vi "Write then read.vi"(7 "error in (no error)":errorcluster, 9 "TX Data":string, 10 "Motor_Serial in":refnum<class "Serial.lvclass">) -> (0 "error out":errorcluster, 2 "RX Data":i32, 3 "Motor_Serial out":refnum<class "Serial.lvclass">)   [LabVIEW 2019, in "Serial.lvclass"]
uses:
  Serial.lvclass
  Serial.lvclass/Serial.ctl
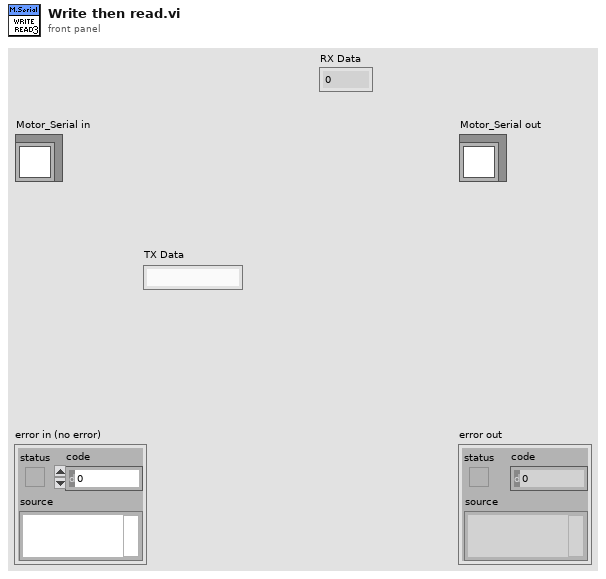
[diagram p1: front panel]
types:
  T1 = typedef "Semaphore RefNum" = refnum<k1>
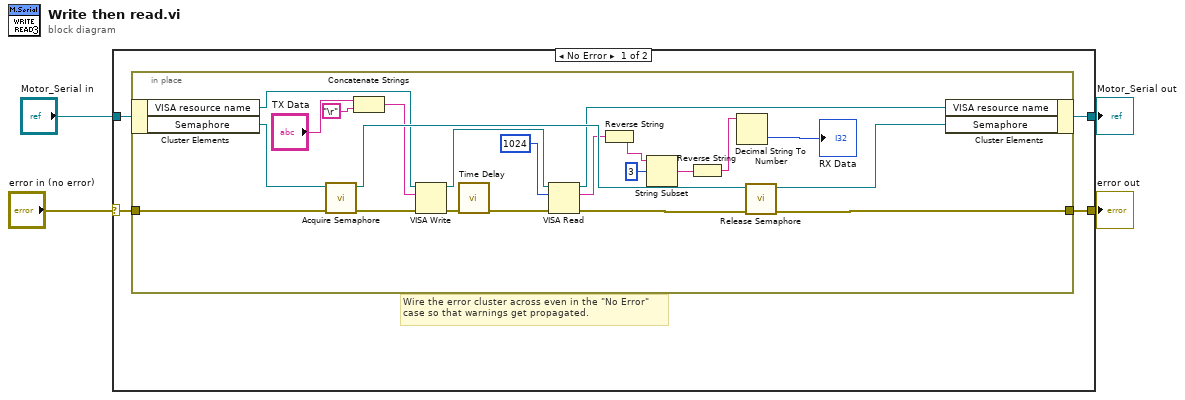
[diagram p0: block diagram]
diagram:
  n1 = case shown="No Error" "error in (no error)" {
    selector: "error in (no error)" -> [w8 w32]
    tunnel: [w7 w32] -> w3
    tunnel: [w5 w31] -> w1
    tunnel: "Motor_Serial in" -> [w6 w31]
    frame No Error {
      # "Wire the error cluster across even in the \"No Error\"\ncase so that warnings get propagated."
      n2 = in-place {
        in-place-border: w8 -> [w22]
        in-place-border: [w21] -> w7
        n3 = in-place-cluster #1(w6) -> ("VISA resource name"=w24:refnum<visa-resource-name>, "Semaphore"=w25:T1)
        n4 = call <vilib>:"Acquire Semaphore.vi"("error in (no error)"=w22, "semaphore"=w25) -> ("error out"=w29:errorcluster, "semaphore out"=w30:T1)  [unwired: 3 in, 1 out]
        n5 = Concatenate Strings("TX Data", "\r") -> (w28:string)
        n6 = VISA Write(VISA resource name=w24, write buffer=w28, error in (no error)=w29) -> (VISA resource name out=w17:refnum<visa-resource-name>, error out=w26:errorcluster)  [unwired: 1 out]
        n7 = call "Time Delay"("error in (no error)"=w26) -> ("error out"=w19:errorcluster)  [unwired: 10 in]
        n8 = VISA Read(VISA resource name=w17, byte count=u32 1024, error in (no error)=w19) -> (VISA resource name out=w15:refnum<visa-resource-name>, read buffer=w10:string, error out=w18:errorcluster)  [unwired: 1 out]
        n9 = Reverse String(1:w10) -> (0:w13:string)
        n10 = String Subset(string=w13, offset (0)=3) -> (substring=w12:string)  [unwired: 1 in]
        n11 = Reverse String(1:w12) -> (0:w11:string)
        n12 = Decimal String To Number(string=w11) -> (number=→"RX Data":i32)  [unwired: 2 in, 1 out]
        n13 = call <vilib>:"Release Semaphore.vi"("error in (no error)"=w18, "semaphore"=w30) -> ("error out"=w21:errorcluster, "semaphore out"=w23:T1)  [unwired: 4 in]
        n14 = in-place-cluster #1("VISA resource name"=w15, "Semaphore"=w23) -> (w5:refnum<class "Serial.lvclass">)
      }
    }
    frame Error {
    }
  }
  "error out" <- w3
  "Motor_Serial out" <- w1
